vi "initalInterpreter.vi"() -> (0 "错误输出":errorcluster caption="error out", 1 "lua_State *print thread":u64, 2 "lua_State *commandthread":u64, 3 "lua_State *mainthread":u64, 4 "printoccur":i32, 5 "readoccur":i32, 7 "writeoccur":i32)   [LabVIEW 2011]
panel:
  out "lua_type":i32(ring) items=["LUA_TNONE"=-1, "LUA_TNIL"=0, "LUA_TBOOLEAN"=1, "LUA_TLIGHTUSERDATA"=2, "LUA_TNUMBER "=3, "LUA_TSTRING"=4, "LUA_TTABLE"=5, "LUA_TFUNCTION"=6, "LUA_TUSERDATA"=7, "LUA_TTHREAD"=8, "LUA_NUMTAGS "=9]
  out "lua_gettop":i32
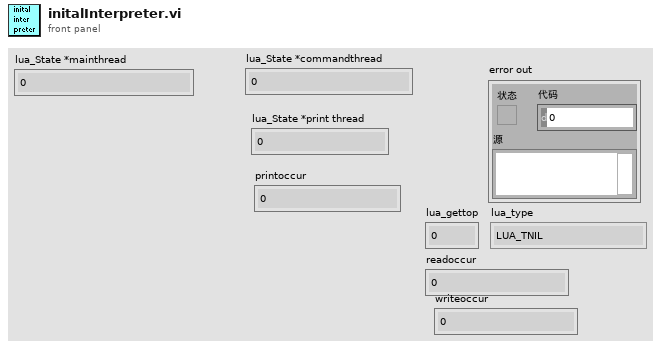
[diagram p1: front panel]
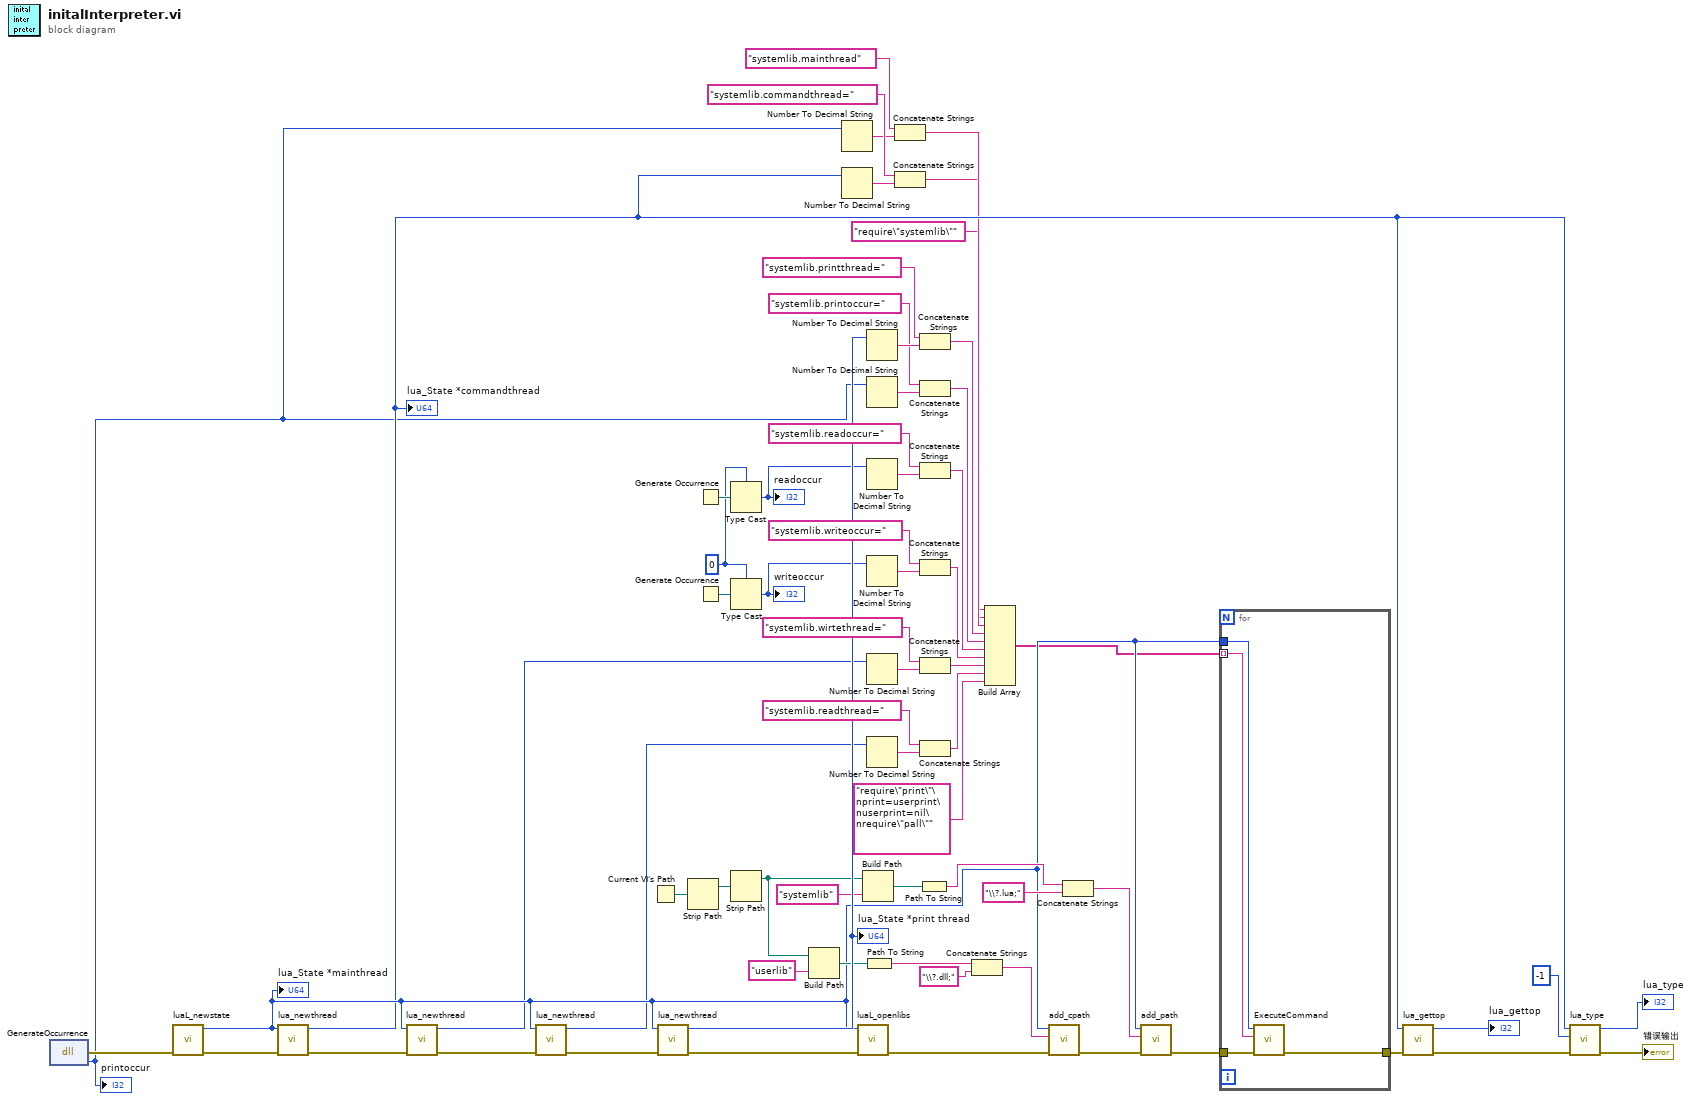
[diagram p0: block diagram]
diagram:
  w36 = 0 ("返回类型")
  n1 = dll-call lib="PTH1}abs GMy DBank\t_work_panmonkey task 2012source programLuaDllToLabviewbuilds\ttestC_dll\t我的DLLOccurrence.dll" fn="GenerateOccurrence"() -> (error out=w65:errorcluster, "返回类型"=w4:i32)  [unwired: 3 in, 1 out]
  "printoccur" <- w4
  n2 = call "luaL_newstate.vi"("error in"=w65) -> ("error out"=w66:errorcluster, "lua_State *luaL_newstate"=w20:u64)  [unwired: 9 in]
  "lua_State *mainthread" <- w20
  n3 = call "lua_newthread.vi"("error in"=w66, "lua_State *L"=w20) -> ("error out"=w21:errorcluster, "lua_State *lua_newthread"=w5:u64)  [unwired: 8 in]
  "lua_State *commandthread" <- w5
  n4 = call "lua_newthread.vi"("error in"=w21, "lua_State *L"=w20) -> ("error out"=w23:errorcluster, "lua_State *lua_newthread"=w19:u64)  [unwired: 8 in]
  n5 = call "lua_newthread.vi"("error in"=w23, "lua_State *L"=w20) -> ("error out"=w22:errorcluster, "lua_State *lua_newthread"=w18:u64)  [unwired: 8 in]
  n6 = Current VI's Path() -> (path=w48:path)
  n7 = call "lua_newthread.vi"("error in"=w22, "lua_State *L"=w20) -> ("error out"=w43:errorcluster, "lua_State *lua_newthread"=w64:u64)  [unwired: 8 in]
  "lua_State *print thread" <- w64
  n8 = Strip Path(path=w48) -> (stripped path=w47:path)  [unwired: 1 out]
  n9 = Generate Occurrence() -> (w38:refnum<k4>)
  n10 = Generate Occurrence() -> (w37:refnum<k4>)
  n11 = Type Cast(type=w36, x=w38) -> (*(type *) &x=w35:i32)
  "readoccur" <- w35
  n12 = Type Cast(type=w36, x=w37) -> (*(type *) &x=w34:i32)
  "writeoccur" <- w34
  n13 = Strip Path(path=w47) -> (stripped path=w56:path)  [unwired: 1 out]
  n14 = Build Path(base path=w56, name or relative path="userlib" ("名称或相对路径")) -> (appended path=w58:path)
  n15 = Number To Decimal String(number=w4) -> (decimal integer string=w7:string)  [unwired: 1 in]
  n16 = Number To Decimal String(number=w5) -> (decimal integer string=w8:string)  [unwired: 1 in]
  n17 = call "luaL_openlibs.vi"("error in"=w43, "lua_State *L"=w20) -> ("error out"=w44:errorcluster)  [unwired: 9 in]
  n18 = Build Path(base path=w56, name or relative path="systemlib" ("名称或相对路径")) -> (appended path=w50:path)
  n19 = Path To String(path=w58) -> (string=w59:string)
  n20 = Number To Decimal String(number=w64) -> (decimal integer string=w63:string)  [unwired: 1 in]
  n21 = Number To Decimal String(number=w4) -> (decimal integer string=w60:string)  [unwired: 1 in]
  n22 = Number To Decimal String(number=w35) -> (decimal integer string=w32:string)  [unwired: 1 in]
  n23 = Number To Decimal String(number=w34) -> (decimal integer string=w30:string)  [unwired: 1 in]
  n24 = Number To Decimal String(number=w19) -> (decimal integer string=w26:string)  [unwired: 1 in]
  n25 = Number To Decimal String(number=w18) -> (decimal integer string=w24:string)  [unwired: 1 in]
  n26 = Concatenate Strings("systemlib.mainthread" ("字符串"), w7) -> (w3:string)
  n27 = Concatenate Strings("systemlib.commandthread=" ("字符串"), w8) -> (w2:string)
  n28 = Path To String(path=w50) -> (string=w54:string)
  n29 = Concatenate Strings("systemlib.printthread=" ("字符串"), w63) -> (w16:string)
  n30 = Concatenate Strings("systemlib.printoccur=" ("字符串"), w60) -> (w15:string)
  n31 = Concatenate Strings("systemlib.readoccur=" ("字符串"), w32) -> (w14:string)
  n32 = Concatenate Strings("systemlib.writeoccur=" ("字符串"), w30) -> (w13:string)
  n33 = Concatenate Strings("systemlib.wirtethread=" ("字符串"), w26) -> (w12:string)
  n34 = Concatenate Strings("systemlib.readthread=" ("字符串"), w24) -> (w11:string)
  n35 = Concatenate Strings(w59, "\\?.dll;" ("字符串")) -> (w52:string)
  n36 = Build Array("require\"systemlib\"", w2, w3, w16, w15, w14, w13, w12, w11, "require\"print\"\nprint=userprint\nuserprint=nil\nrequire\"pall\"") -> (w17:string[])
  n37 = call "add_cpath.vi"("error in"=w44, "string"=w52, "lua_State *L"=w20) -> ("error out"=w45:errorcluster)  [unwired: 8 in]
  n38 = Concatenate Strings(w54, "\\?.lua;" ("字符串")) -> (w55:string)
  n39 = call "add_path.vi"("error in"=w45, "string"=w55, "lua_State *L"=w20) -> ("error out"=w29:errorcluster)  [unwired: 8 in]
  n40 = for {
    tunnel: w29 -> [w70]
    tunnel: [w69] -> w28
    tunnel: w20 -> [w68]
    tunnel: w17 -> [w67] mode=indexing
    n41 = call "ExecuteCommand.vi"("error in"=w70, "command(ctrl+enter)"=w67, "lua_State *luaL_newstate"=w68) -> ("error out"=w69:errorcluster)  [unwired: 6 in, 2 out]
  }
  n42 = call "lua_gettop.vi"("error in"=w28, "lua_State *L"=w5) -> ("error out"=w42:errorcluster, "lua_gettop"=→"lua_gettop":i32)  [unwired: 8 in]
  n43 = call "lua_type.vi"("error in"=w42, "int index"=-1, "lua_State *L"=w5) -> ("error out"=→"错误输出":errorcluster, "lua_type"=→"lua_type":i32)  [unwired: 7 in]
